vi "demo - first VI with defaults.vi"() -> ()   [LabVIEW 2024]
panel:
  out "Temperature History":dbl(graph)
  in  "stop":bool
  out "Alarm":bool
  in  "current temperature":dbl
  in  "threshold":dbl
  # "Input"
  # "Output"
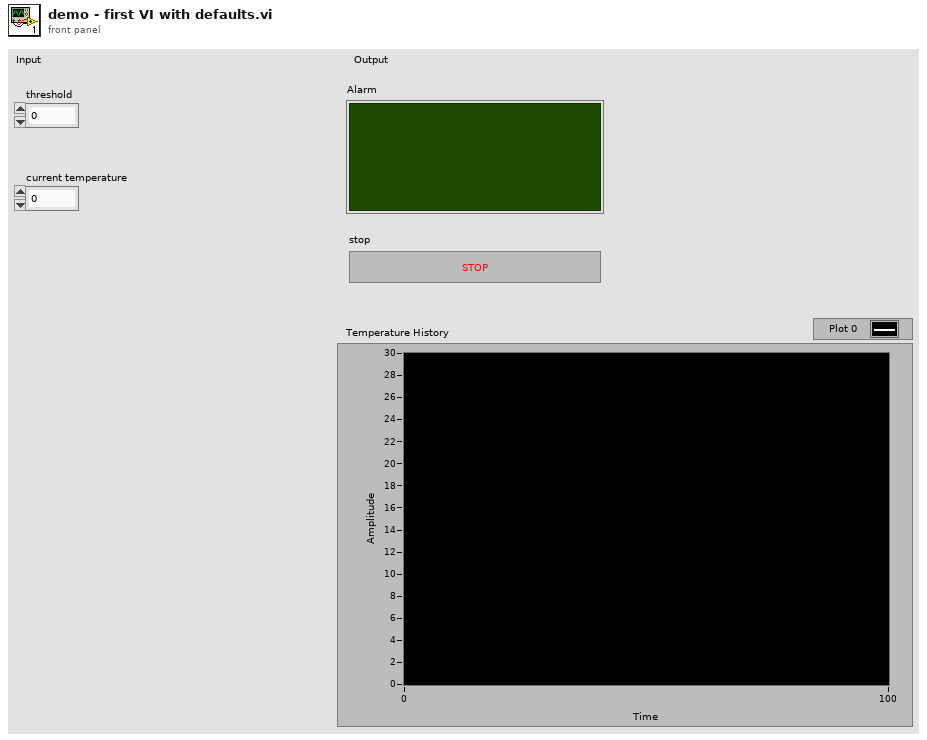
[diagram p1: front panel]
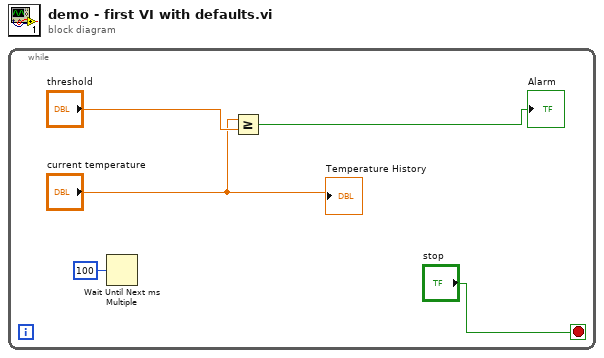
[diagram p0: block diagram]
diagram:
  n1 = while {
    stop <- "stop" stop-if-true
    n2 = Wait Until Next ms Multiple(millisecond multiple=u32 100) -> ()  [unwired: 1 out]
    n3 = Greater Or Equal?(x="current temperature", y="threshold") -> (x >= y?=→"Alarm":bool)
    "Temperature History" <- "current temperature"
  }
